vi "LoadLastLoadedFile.vi"(0 "SetValueInfo in":refnum<vi>[](array[refnum]), 1 "DIMControSet in":refnum<vi>[](array[refnum]), 3 "Data":string, 4 "No Link?":bool, 5 "GUIName":string, 8 "PanelLocation":path, 9 "ListOfBases_Data":refnum<vi>) -> (19 "error out":errorcluster)   [LabVIEW 2014, in "Panels.lvlib"]
uses:
  Panels.lvlib
  CS_Core/CSSystem/CoreDefs/CoreDefs.call_type.ctl
  CS_Core/BaseProcess/BaseProcess.descriptor string definition.ctl
  CS_Core/CSSystem/CoreDefs/CoreDefs.rawDataType.ctl
  CS_Core/CSSystem/CoreLib/CoreLib.string 2 byte array.vi
  CS_Core/CSSystem/CoreLib/CoreLib.short 2 byte array.vi
  CS_Core/CSSystem/CoreLib/CoreLib.lvlib
  CS_Core/BaseProcess/BaseProcess.lvlib
panel:
  in  "call cluster in":T1={"Object"="", "Selector"="", "CallType"=enum."synchronous", "Async Object"="", "Async Selector"="", "Data Descriptor"="", "Data"=[], "Error #"=0, "Expire"=0}
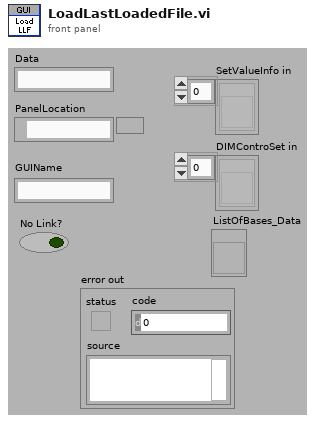
[diagram p1: front panel]
types:
  T1 = typedef "CoreDefs.call_type.ctl" = cluster{"Object":string, "Selector":string, "CallType":enum16{"simple", "synchronous", "asynchronous"}, "Async Object":string, "Async Selector":string, "Data Descriptor":T2, "Data":T3, "Error #":i32, "Expire":u32}
  T2 = typedef "BaseProcess.lvlib/BaseProcess.descriptor string definition.ctl" = string
  T3 = typedef "CoreDefs.rawDataType.ctl" = i8[]
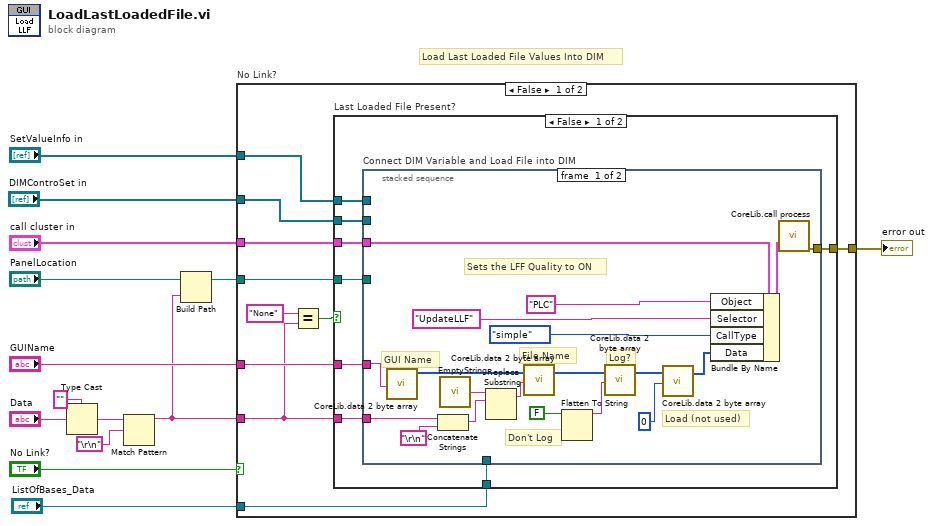
[diagram p0: block diagram]
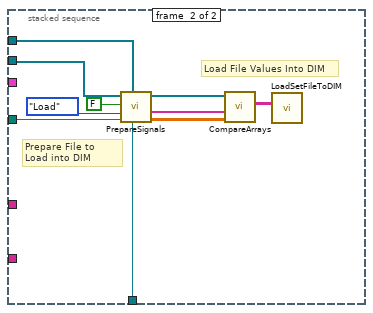
[diagram p2: hidden frame]
diagram:
  # "Load Last Loaded File Values Into DIM"
  n1 = Type Cast(type="" ("regular expression"), x="Data") -> (*(type *) &x=w9:string)
  n2 = Match Pattern(string=w9, regular expression="\r\n") -> (before substring=w6:string)  [unwired: 1 in, 3 out]
  n3 = Build Path(base path="PanelLocation", name or relative path=w6) -> (appended path=w7:path)
  n4 = case "No Link?" shown="False" "No Link?" {
    tunnel: "GUIName" -> [w19 _]
    tunnel: "call cluster in" -> [w24 _]
    tunnel: "DIMControSet in" -> [w23 _]
    tunnel: w7 -> [w22 _]
    tunnel: w6 -> [w17 _]
    tunnel: [w21 _] -> w5
    tunnel: "SetValueInfo in" -> [w16 _]
    tunnel: "ListOfBases_Data" -> [w15 _]
    frame False {
      n5 = Equal?(x="None", y=w17) -> (x = y?=w20:bool)
      n6 = case "Last Loaded File Present?" shown="False" w20 {
        tunnel: w24 -> [w32 _]
        tunnel: w19 -> [w31 _]
        tunnel: w17 -> [w30 _]
        tunnel: w23 -> [w29 _]
        tunnel: w22 -> [w28 _]
        tunnel: [w27 _] -> w21
        tunnel: w16 -> [w26 _]
        tunnel: w15 -> [w25 _]
        frame False {
          n7 = stacked-sequence "Connect DIM Variable and Load File into DIM" {
            tunnel: w32 -> [w42 _]
            tunnel: w31 -> [w41 _]
            tunnel: w30 -> [w39 _]
            tunnel: w29 -> [_ w58]
            tunnel: w28 -> [_ w56]
            tunnel: [w40 _] -> w27
            tunnel: w26 -> [_ w53]
            tunnel: w25 -> [_ w52]
            frame #0 {
              # "Load (not used)"
              # "Log?"
              # "File Name"
              # "GUI Name"
              # "Don't Log"
              # "Sets the LFF Quality to ON"
              n8 = call-poly "CoreLib.data 2 byte array.vi"("string"=w41) -> ("byteArray out"=w47:T3)  [unwired: 18 in]
              n9 = Concatenate Strings(w39, "\r\n") -> (w43:string)
              n10 = call "EmptyString.vi"() -> ("String"=w46:string)
              n11 = Replace Substring(4:w43, 5:w46) -> (1:w44:string)  [unwired: 2 in, 1 out]
              n12 = call-poly "CoreLib.data 2 byte array.vi"("byteArray"=w47, "string"=w44) -> ("byteArray out"=w37:T3)  [unwired: 17 in]
              n13 = Flatten To String(anything=FALSE) -> (data string=w36:string)  [unwired: 3 in, 2 out]
              n14 = call-poly "CoreLib.data 2 byte array.vi"("byteArray"=w37, "string"=w36) -> ("byteArray out"=w35:T3)  [unwired: 17 in]
              n15 = call-poly "CoreLib.data 2 byte array.vi"("byteArray"=w35, "i16"=i16 0) -> ("byteArray out"=w34:T3)  [unwired: 17 in]
              n16 = Bundle By Name(cluster=w42, "Object"="PLC", "Selector"="UpdateLLF" ("serviceName"), "CallType"=enum16{"simple", "synchronous", "asynchronous"}."simple", "Data"=w34) -> (w51:T1)
              n17 = call "CoreLib.call process.vi"("call cluster in"=w51) -> ("error out"=w40:errorcluster)  [unwired: 13 in, 1 out]
            }
            frame #1 {
              # "Load File Values Into DIM"
              # "Prepare File to Load into DIM"
              n18 = call "PrepareSignals.vi"("ListOfBases_Data"=w52, "SetValueInfo in"=w53, "setfile path"=w56, "Enum"=enum16{"Save", "Load"}."Load", "Display Message to \nUser"=FALSE ("Display Message to \nUser"), "DIMControSet in"=w58) -> ("indexed loaded Array"=w61:dbl[][], "Name Array"=w60:string[], "DIMControSet out"=w59:refnum<vi>[])  [unwired: 3 in]
              n19 = call "CompareArrays.vi"("indexed loaded Array"=w61, "Name Array"=w60, "DIMControSet"=w59) -> ("Table for loading values"=w55:string[][])  [unwired: 4 in]
              n20 = call "LoadSetFileToDIM.vi"("output array"=w55) -> ()  [unwired: 2 in]
            }
          }
        }
        frame True {
        }
      }
    }
    frame True {
    }
  }
  "error out" <- w5
